vi "ExecuteMenuCommand.vi"(0 "reference in":refnum<class "DQMHModuleNode.lvclass">, 1 "Command":string, 5 "error in (no error)":errorcluster) -> (14 "reference out":refnum<class "DQMHModuleNode.lvclass">, 15 "EditorAction":T3, 16 "FlattenCommandSettings":T1, 19 "error out":errorcluster)   [LabVIEW 2016, in "DQMHModuleNode.lvclass"]
uses:
  <resource>/Framework/Providers/Open_GDS/UML/DQMHModuleNode_class/DQMHModuleNode.lvclass
  <resource>/Framework/Providers/Open_GDS/UML/UMLEditor/UMLEditor EditorActionType.ctl
  <resource>/Framework/Providers/Open_GDS/UML/UMLEditor/UMLEditor FlattenCommandType.ctl
  <resource>/Framework/Providers/Open_GDS/UML/UMLEditor/UMLEditor ExecuteCommandType.ctl
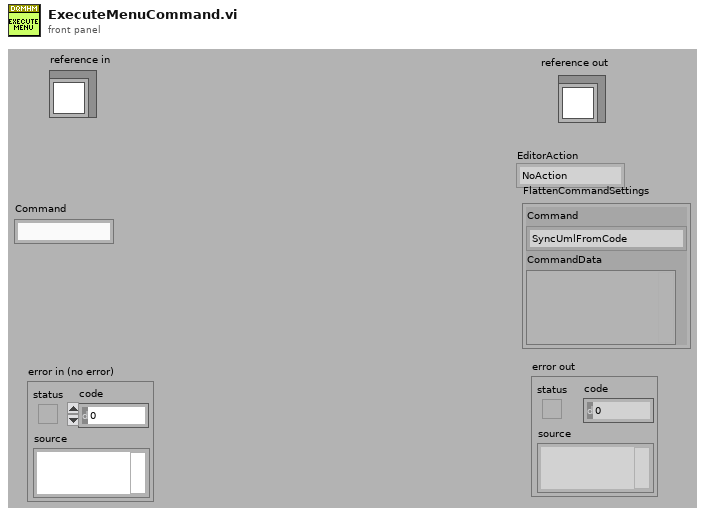
[diagram p1: front panel]
types:
  T1 = typedef "UMLEditor FlattenCommandType.ctl" = cluster{"Command":T2, "CommandData":variant}
  T2 = typedef "UMLEditor ExecuteCommandType.ctl" = enum16{"SyncUmlFromCode", "SyncCodeFromUML", "OpenClass", "OpenFile", "CreateClass", "CreateVI", "OpenClassAttribute", "LocateInProject", "GraphExecute"}
  T3 = typedef "UMLEditor EditorActionType.ctl" = enum16{"NoAction", "Repaint", "ExecuteCommand"}
  T4 = typedef "DQMHModuleNode.lvclass/ObjectAttributes.ctl" = cluster{"DescriptionHeight":dbl, "InternalDataHeight":dbl, "EventsHeight":dbl, "Name":refnum<class "MultiLineString.lvclass">, "Description":refnum<class "MultiLineString.lvclass">, "InternalData":refnum<class "MultiLineString.lvclass">, "Events":refnum<class "MultiLineString.lvclass">, "showDescription":bool, "showInternalData":bool, "showEvents":bool, "DEFAULT_ROUNDING":i32, "DEFAULT_WIDTH":i32, "DEFAULT_HEIGHT":i32, "ClassPath":path, "Template":string, "Icon":u8[][]}
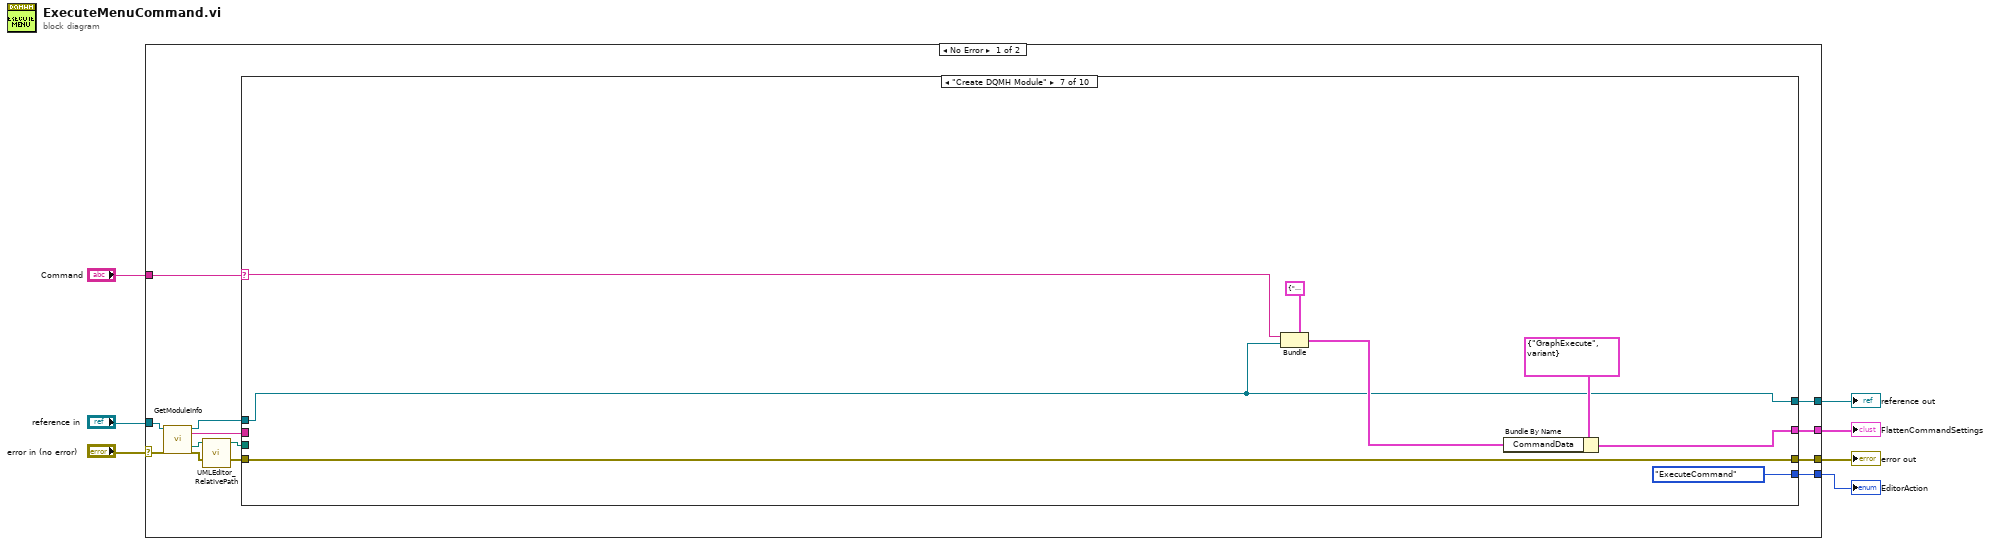
[diagram p0: block diagram]
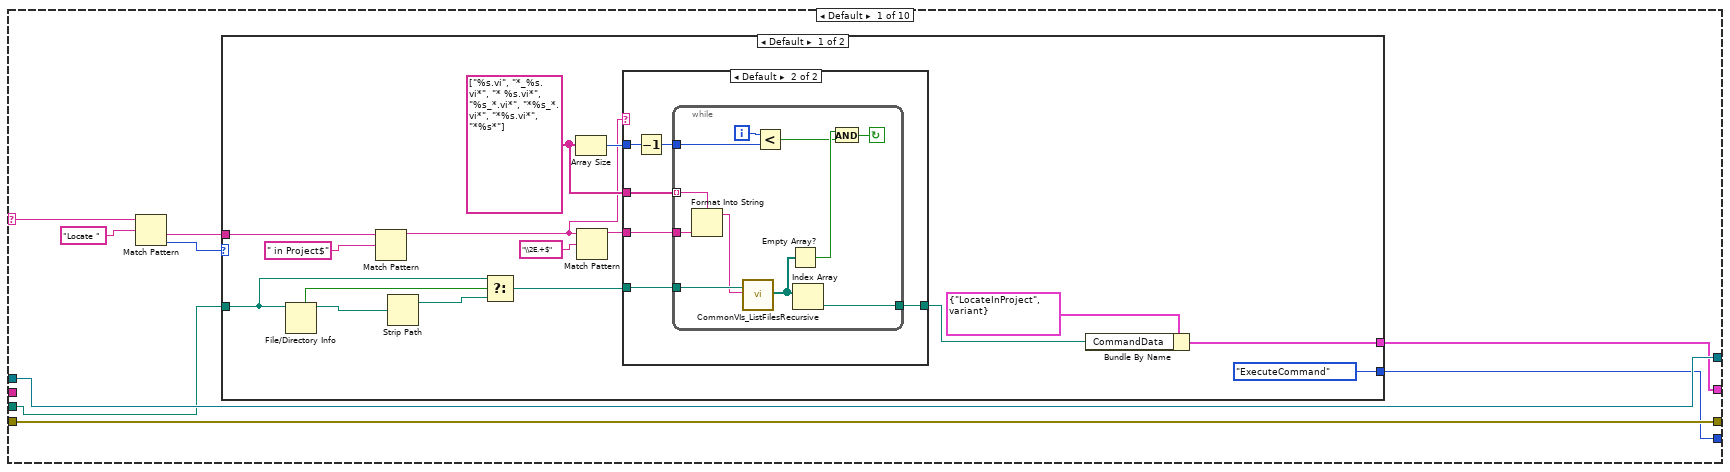
[diagram p2: hidden frame]
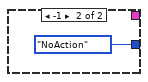
[diagram p4: hidden frame]
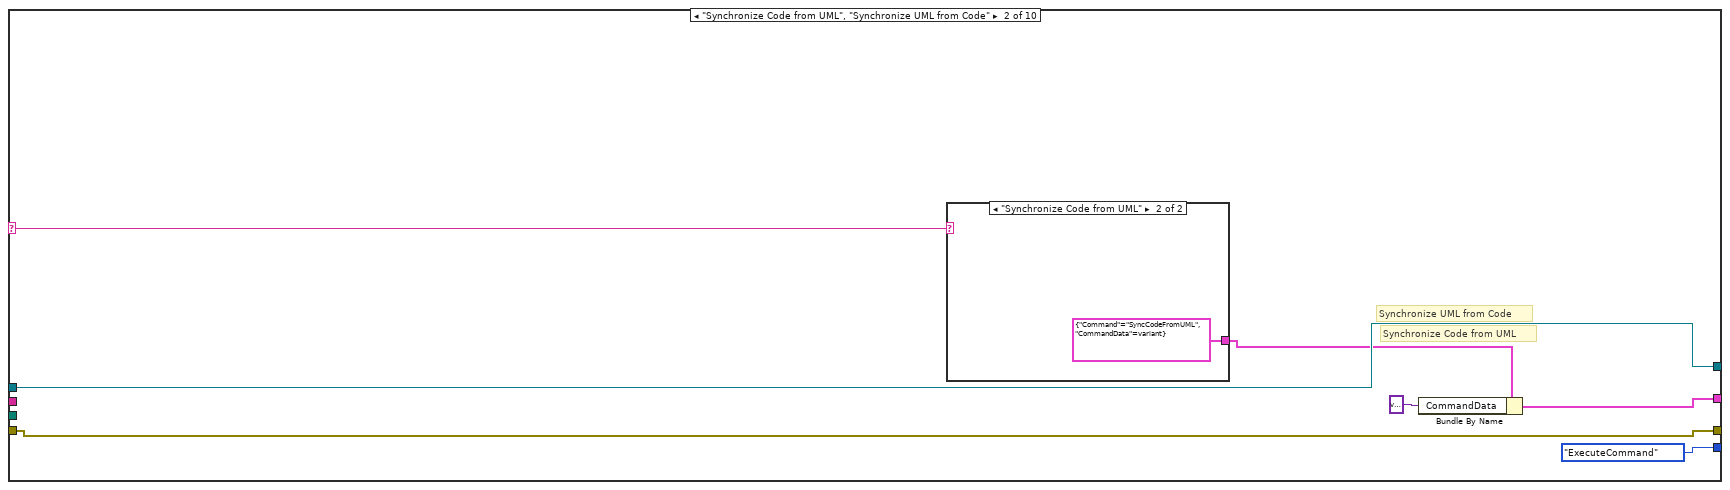
[diagram p5: hidden frame]
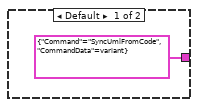
[diagram p6: hidden frame]
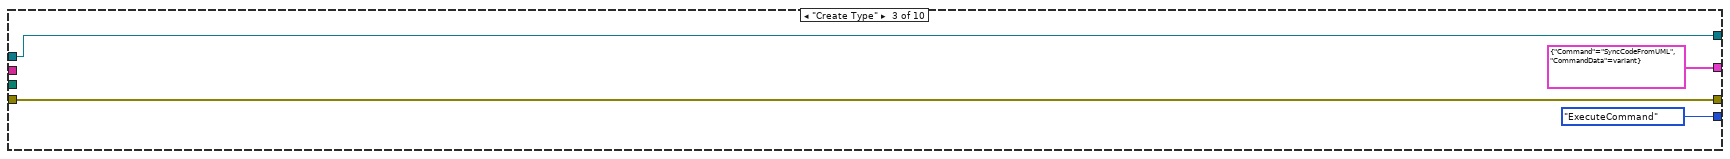
[diagram p7: hidden frame]
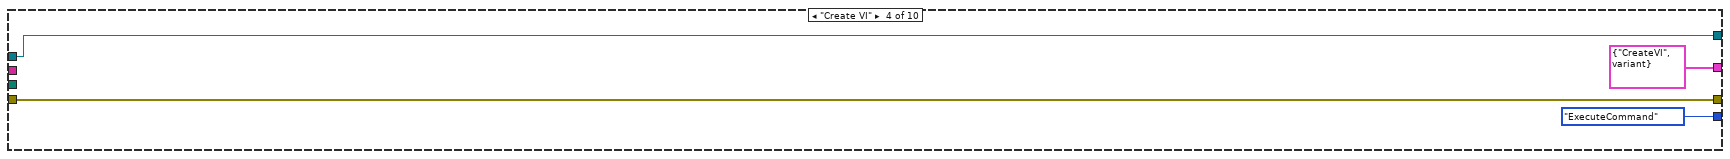
[diagram p8: hidden frame]
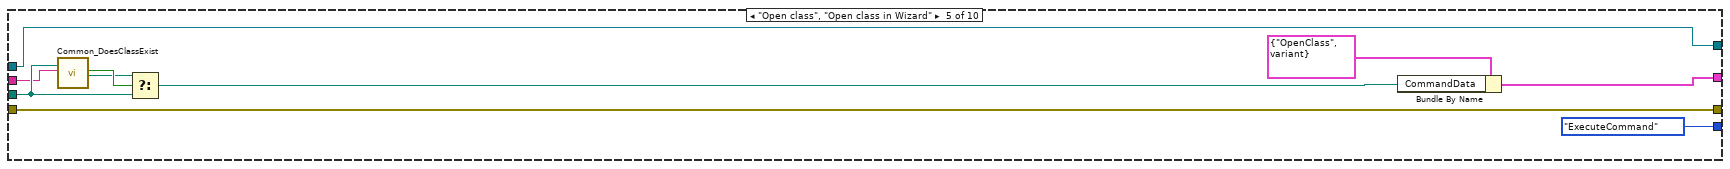
[diagram p9: hidden frame]
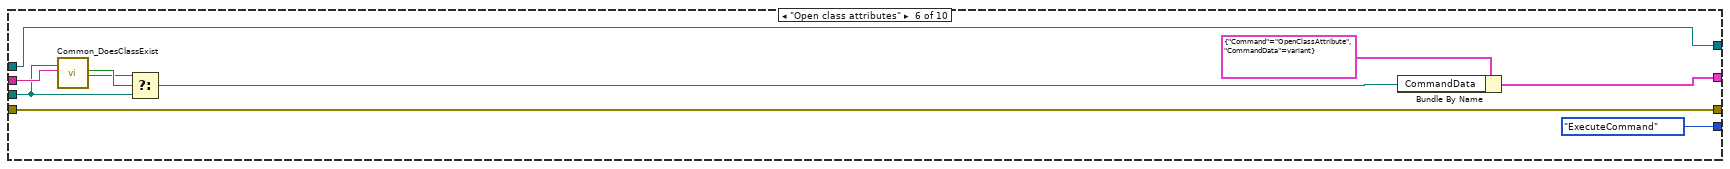
[diagram p10: hidden frame]
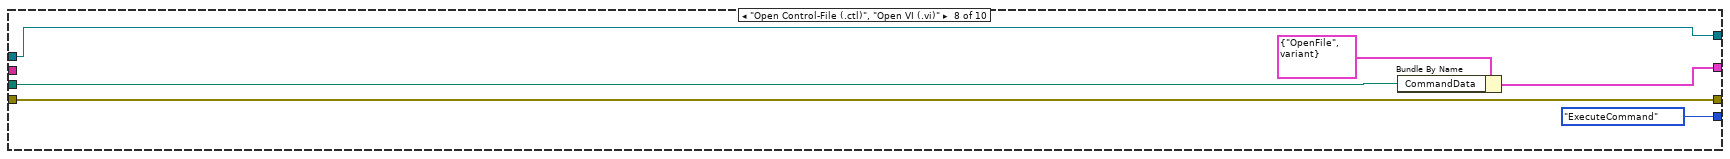
[diagram p11: hidden frame]
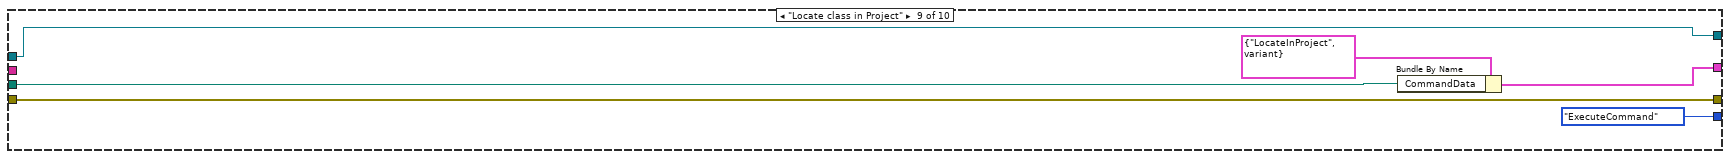
[diagram p12: hidden frame]
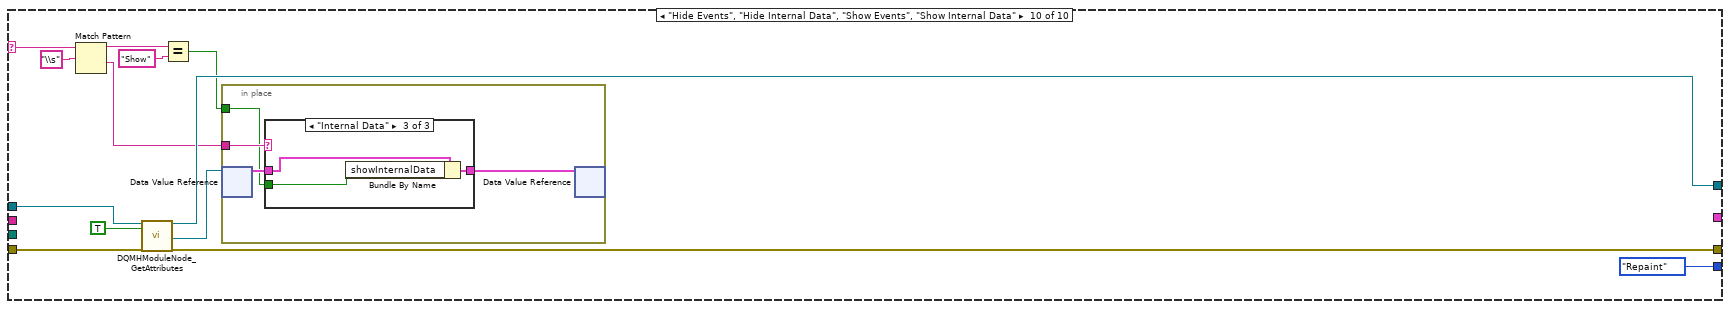
[diagram p13: hidden frame]
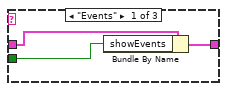
[diagram p14: hidden frame]
diagram:
  n1 = case shown="No Error" "error in (no error)" {
    selector: "error in (no error)" -> [w12 w144]
    tunnel: "reference in" -> [w14 w145]
    tunnel: [w17 w144] -> w5
    tunnel: [w18 w145] -> w4
    tunnel: "Command" -> [w19 _]
    tunnel: [w16 _] -> w2
    tunnel: [w15 _] -> w1
    frame No Error {
      n2 = call-dynamic "GetModuleInfo.vi"("reference in"=w14, "error in (no error)"=w12) -> ("reference out"=w13:refnum<class "DQMHModuleNode.lvclass">, "ModuleName"=w10:string, "ModulePath"=w9:path, "error out"=w11:errorcluster)  [unwired: 6 in, 8 out]
      n3 = call <resource>:"UMLEditor_RelativePath.vi"("Path In"=w9) -> ("ConvertToAbsolutePath(If possible)"=w8:path)  [unwired: 1 in, 17 out]
      n4 = case shown="\"Create DQMH Module\"" w19 {
        selector: w19 -> [w25 w63 _ _ _ _ w102 _ _ w127]
        tunnel: w11 -> [w27 w67 w72 w76 w87 w90 w106 w111 w117 w129]
        tunnel: w13 -> [w28 w68 w73 w77 w88 w98 w100 w112 w118 w131]
        tunnel: [w28 w68 w73 w77 w88 w98 w100 w112 w118 w130] -> w18
        tunnel: [w27 w67 w72 w76 w87 w90 w106 w111 w117 w128] -> w17
        tunnel: [w26 UMLEditor_EditorActionType."ExecuteCommand" ("EditorAction") UMLEditor_EditorActionType."ExecuteCommand" ("EditorAction") UMLEditor_EditorActionType."ExecuteCommand" ("EditorAction") UMLEditor_EditorActionType."ExecuteCommand" ("EditorAction") UMLEditor_EditorActionType."ExecuteCommand" ("EditorAction") UMLEditor_EditorActionType."ExecuteCommand" ("EditorAction") UMLEditor_EditorActionType."ExecuteCommand" ("EditorAction") UMLEditor_EditorActionType."ExecuteCommand" ("EditorAction") UMLEditor_EditorActionType."Repaint" ("EditorAction")] -> w16
        tunnel: [w21 w65 T1 {"Command"=enum."SyncCodeFromUML", "CommandData"=variant} ("FlattenCommandSettings") T1 {"Command"=enum."CreateVI", "CommandData"=variant} ("FlattenCommandSettings") w85 w96 w104 w109 w115 _] -> w15
        tunnel: w8 -> [w20 _ _ _ w81 w91 _ w108 w114 _]
        tunnel: w10 -> [_ _ _ _ w80 w92 _ _ _ _]
        frame Default {
          n5 = Match Pattern(string=w25, regular expression="Locate ") -> (after substring=w22:string, offset past match=w23:i32)  [unwired: 1 in, 2 out]
          n6 = case shown="Default" w23 {
            tunnel: [UMLEditor_EditorActionType."ExecuteCommand" ("EditorAction") UMLEditor_EditorActionType."NoAction" ("EditorAction")] -> w26
            tunnel: w22 -> [w44 _]
            tunnel: [w40 _] -> w21
            tunnel: w20 -> [w30 _]
            frame Default {
              w35 = string[] ["%s.vi", "*_%s.vi*", "* %s.vi*", "%s_*.vi*", "*%s_*.vi*", "*%s.vi*", "*%s*"]
              n7 = File/Directory Info(path=w30) -> (path out=w33:path, directory=w38:bool)  [unwired: 1 in, 5 out]
              n8 = Match Pattern(string=w44, regular expression=" in Project$") -> (before substring=w31:string)  [unwired: 1 in, 3 out]
              n9 = Strip Path(path=w33) -> (stripped path=w32:path)  [unwired: 1 out]
              n10 = Select(t=w30, s=w38, f=w32) -> (s? t:f=w37:path)
              n11 = Array Size(array=w35) -> (size(s)=w34:i32)
              n12 = Match Pattern(string=w31, regular expression="\\2E.+$") -> (before substring=w36:string)  [unwired: 4 out]
              n13 = case shown="Default" w31 {
                tunnel: [_ w47] -> w29
                tunnel: w37 -> [_ w50]
                tunnel: w35 -> [_ w49]
                tunnel: w36 -> [_ w48]
                tunnel: w34 -> [_ w46]
                frame "" {
                }
                frame Default {
                  n14 = Decrement(x=w46) -> (x-1=w45:i32)
                  n15 = while {
                    tunnel: w50 -> [w61]
                    tunnel: w49 -> [w60] mode=indexing
                    tunnel: w48 -> [w59]
                    tunnel: [w58] -> w47
                    tunnel: w45 -> [w54]
                    i -> [w55]
                    stop <- w51 continue-if-true
                    n16 = Format Into String(format string=w60, w59) -> (resulting string=w56:string)  [unwired: 2 in, 1 out]
                    n17 = call <resource>:"CommonVIs_ListFilesRecursive.vi"("directory path"=w61, "FileSearchPattern"=w56) -> ("Files"=w57:path[])  [unwired: 4 in, 13 out]
                    n18 = Less?(x=w55, y=w54) -> (x < y?=w52:bool)
                    n19 = Empty Array?(array=w57) -> (empty?=w53:bool)
                    n20 = Index Array(array=w57) -> (element=w58:path)  [unwired: 1 in]
                    n21 = And(x=w53, y=w52) -> (x .and. y?=w51:bool)
                  }
                }
              }
              n22 = Bundle By Name(cluster=T1 {"Command"=enum."LocateInProject", "CommandData"=variant} ("FlattenCommandSettings"), "CommandData"=w29) -> (w40:T1)
            }
            frame -1 {
            }
          }
        }
        frame "Synchronize Code from UML", "Synchronize UML from Code" {
          # "Synchronize Code from UML"
          # "Synchronize UML from Code"
          n23 = case shown="\"Synchronize Code from UML\"" w63 {
            tunnel: [T1 {"Command"=enum."SyncUmlFromCode", "CommandData"=variant} ("FlattenCommandSettings") T1 {"Command"=enum."SyncCodeFromUML", "CommandData"=variant} ("FlattenCommandSettings")] -> w66
            frame Default {
            }
            frame "Synchronize Code from UML" {
            }
          }
          n24 = Bundle By Name(cluster=w66, "CommandData"=variant) -> (w65:T1)
        }
        frame "Create Type" {
        }
        frame "Create VI" {
        }
        frame "Open class", "Open class in Wizard" {
          n25 = call <resource>:"Common_DoesClassExist.vi"("ClassPath"=w81, "ClassName"=w80) -> ("llb-class"=w83:bool, "llb/LvCLass-Path"=w82:path)  [unwired: 16 out]
          n26 = Select(t=w82, s=w83, f=w81) -> (s? t:f=w84:path)
          n27 = Bundle By Name(cluster=T1 {"Command"=enum."OpenClass", "CommandData"=variant} ("FlattenCommandSettings"), "CommandData"=w84) -> (w85:T1)
        }
        frame "Open class attributes" {
          n28 = call <resource>:"Common_DoesClassExist.vi"("ClassPath"=w91, "ClassName"=w92) -> ("llb-class"=w94:bool, "llb/LvCLass-Path"=w93:path)  [unwired: 16 out]
          n29 = Select(t=w93, s=w94, f=w91) -> (s? t:f=w95:path)
          n30 = Bundle By Name(cluster=T1 {"Command"=enum."OpenClassAttribute", "CommandData"=variant} ("FlattenCommandSettings"), "CommandData"=w95) -> (w96:T1)
        }
        frame "Create DQMH Module" {
          n31 = Bundle(cluster=cluster{"Cmd":string, "Data":variant} {"Cmd"="", "Data"=variant} ("FlattenCommandSettings"), "Cmd"=w102, "Data"=w100) -> (w101:cluster{"Cmd":string, "Data":variant})
          n32 = Bundle By Name(cluster=T1 {"Command"=enum."GraphExecute", "CommandData"=variant} ("FlattenCommandSettings"), "CommandData"=w101) -> (w104:T1)
        }
        frame "Open Control-File (.ctl)", "Open VI (.vi)" {
          n33 = Bundle By Name(cluster=T1 {"Command"=enum."OpenFile", "CommandData"=variant} ("FlattenCommandSettings"), "CommandData"=w108) -> (w109:T1)
        }
        frame "Locate class in Project" {
          n34 = Bundle By Name(cluster=T1 {"Command"=enum."LocateInProject", "CommandData"=variant} ("FlattenCommandSettings"), "CommandData"=w114) -> (w115:T1)
        }
        frame "Hide Events", "Hide Internal Data", "Show Events", "Show Internal Data" {
          n35 = Match Pattern(string=w127, regular expression="\\s") -> (before substring=w123:string, after substring=w121:string)  [unwired: 3 out]
          n36 = call <resource>:"DQMHModuleNode_GetAttributes.vi"("reference in"=w131, "OnlyGetDvrReference(False)"=TRUE, "error in (no error)"=w129) -> ("reference out"=w130:refnum<class "DQMHModuleNode.lvclass">, "DataRef"=w122:refnum<data-value>, "error out"=w128:errorcluster)  [unwired: 13 in, 1 out]
          n37 = Equal?(x=w123, y="Show") -> (x = y?=w120:bool)
          n38 = in-place {
            in-place-border: w121 -> [w136]
            in-place-border: w120 -> [w134]
            n39 = in-place-dvr #1(w122) -> (w135:T4)  [unwired: 1 out]
            n40 = case shown="\"Internal Data\"" w136 {
              tunnel: w135 -> [w139 w140 w143]
              tunnel: [w138 w140 w142] -> w133
              tunnel: w134 -> [w137 _ w141]
              frame "Events" {
                n41 = Bundle By Name(cluster=w139, "showEvents"=w137) -> (w138:T4)
              }
              frame Default {
              }
              frame "Internal Data" {
                n42 = Bundle By Name(cluster=w143, "showInternalData"=w141) -> (w142:T4)
              }
            }
            n43 = in-place-dvr #1(w133) -> ()  [unwired: 2 out]
          }
        }
      }
    }
    frame Error {
    }
  }
  "reference out" <- w4
  "error out" <- w5
  "FlattenCommandSettings" <- w1
  "EditorAction" <- w2
